vi "Create Data Path.vi"(1 "Data Directory Name":string="squeezing") -> (0 "appended path":path)   [LabVIEW 2009]
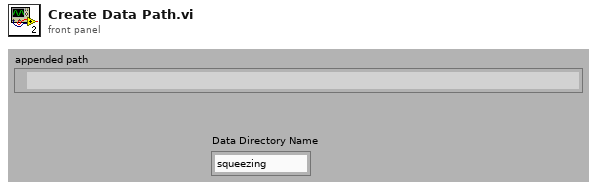
[diagram p1: front panel]
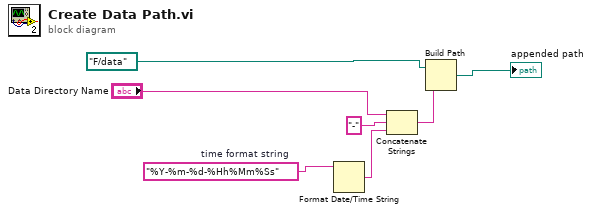
[diagram p0: block diagram]
diagram:
  w3 = "%Y-%m-%d-%Hh%Mm%Ss"  # time format string
  n1 = Format Date/Time String(time format string (%c)=w3) -> (date/time string=w2:string)  [unwired: 2 in]
  n2 = Concatenate Strings("Data Directory Name", "-" ("string"), w2) -> (w4:string)
  n3 = Build Path(base path=path "F:/data" ("Enter Directory"), name or relative path=w4) -> (appended path=→"appended path":path)
